vi "Read Reg.vi"(8 "error in (no error)":errorcluster, 11 "BCReg in":refnum<class "BCReg.lvclass">) -> (0 "error out":errorcluster, 2 "Reg":variant, 3 "BCReg out":refnum<class "BCReg.lvclass">)   [LabVIEW 2014, in "BusController.lvlib" / "BCReg.lvclass"]
uses:
  BCReg.lvclass
  BCReg.lvclass/BCReg.ctl
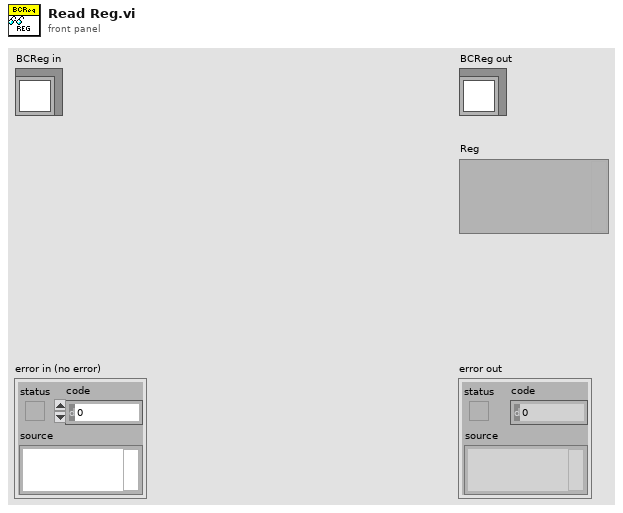
[diagram p1: front panel]
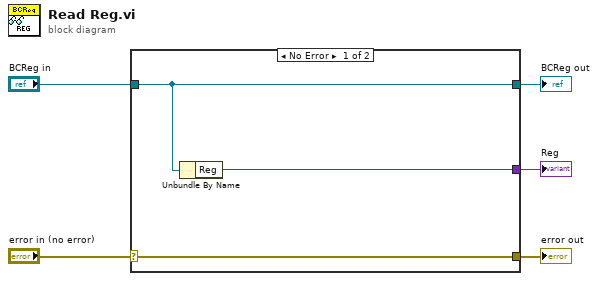
[diagram p0: block diagram]
diagram:
  n1 = case shown="No Error" "error in (no error)" {
    selector: "error in (no error)" -> [w8 w9]
    tunnel: [w8 w9] -> w4
    tunnel: [w7 w10] -> w2
    tunnel: "BCReg in" -> [w7 w10]
    tunnel: [w6 _] -> w1
    frame No Error {
      n2 = Unbundle By Name(w7) -> ("Reg"=w6:variant)
    }
    frame Error {
    }
  }
  "error out" <- w4
  "BCReg out" <- w2
  "Reg" <- w1
